vi "Apply Configuration.vi"(8 "Error In":errorcluster, 11 "reference in":refnum<class "PXIe-5172Ref.lvclass">) -> (0 "Error Out":errorcluster, 3 "reference out":refnum<class "PXIe-5172Ref.lvclass">)   [LabVIEW 2023, in "PXIe-5172.lvlib" / "PXIe-5172Ref.lvclass"]
uses:
  PXIe-5172Ref.lvclass
  PXIe-5172.lvclass
  PXIe-5172Ref.lvclass/PXIe-5172Ref.ctl
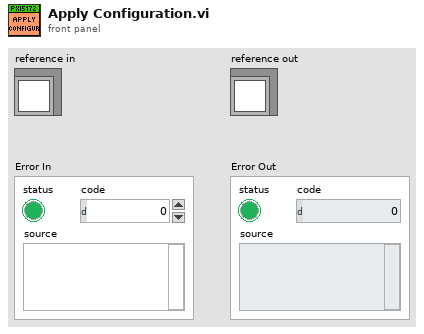
[diagram p1: front panel]
types:
  T1 = typedef "PXIe-5172.lvlib/PXIe-5172Ref.lvclass/ObjectAttributes.ctl" = cluster{"PXIe-5172.lvclass":refnum<class "PXIe-5172.lvclass">}
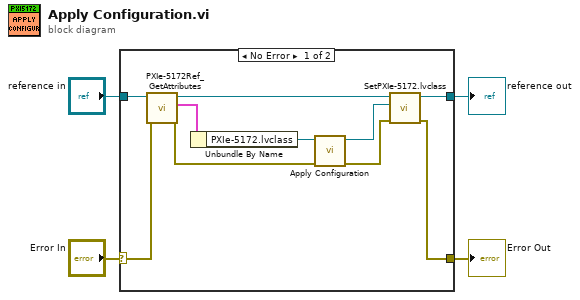
[diagram p0: block diagram]
diagram:
  n1 = case shown="No Error" "Error In" {
    selector: "Error In" -> [w14 w16]
    tunnel: [w6 w16] -> w3
    tunnel: [w8 w15] -> w1
    tunnel: "reference in" -> [w12 w15]
    frame No Error {
      n2 = call "PXIe-5172Ref_GetAttributes.vi"("Error In"=w14, "reference in"=w12) -> ("Error Out"=w9:errorcluster, "Data"=w13:T1, "reference out"=w11:refnum<class "PXIe-5172Ref.lvclass">)  [unwired: 6 in, 1 out]
      n3 = Unbundle By Name(w13) -> ("PXIe-5172.lvclass"=w10:refnum<class "PXIe-5172.lvclass">)
      n4 = call-dynamic "Apply Configuration.vi"("error in"=w9, "Scope Base in"=w10) -> ("error out"=w7:errorcluster, "Scope Base out"=w5:refnum<class "PXIe-5172.lvclass">)  [unwired: 8 in]
      n5 = call "SetPXIe-5172.lvclass.vi"("Error In"=w7, "PXIe-5172.lvclass"=w5, "reference in"=w11) -> ("Error Out"=w6:errorcluster, "reference out"=w8:refnum<class "PXIe-5172Ref.lvclass">)  [unwired: 7 in]
    }
    frame Error {
    }
  }
  "Error Out" <- w3
  "reference out" <- w1
